vi "Acionamento_Adquiri.vi"() -> ()   [LabVIEW 2019]
panel:
  in  "ADQ":bool
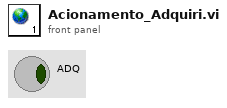
[diagram p1: front panel]
diagram:
